vi "Transform_Calc_b_vector.vi"(9 "C":T1, 10 "PairedFiducialCoordinates":T2[](array[typedef]), 11 "A":T1) -> (3 "b":T1)   [LabVIEW 2011]
doc: "Coordinate system shift to transform reference point to the current coordinate system:\n\nY = A(X-C) + B \n\nWhere X is a point in the refernce system, C is the center of rotation offset to but the first fiducial at the origin for rotation, and A is the rotation and scaling matrix for the tranformation. Y is the coordinate for the point in the current coordinate system and this varialble B is the translation vector.\n\nThis should be approximately the (-1)*Fid_Current_Session(1), ie, the oposite sign of the shift to align the common fiducials for the rotation. Remember C is the shift for the reference session to do the same for it."
uses:
  <vilib>/Analysis/Matrix/Datatypes/RealMatrix.ctl
  Fiducial_pair.ctl
  <vilib>/Analysis/Matrix/Numeric/Conversions/Array To Matrix - RA.vi
  <vilib>/Analysis/Matrix/Numeric/Subtract/Subtract - RM,RM.vi
  <vilib>/Analysis/Matrix/Numeric/Multiply/Multiply - RM,RM.vi
  <vilib>/Analysis/Matrix/Numeric/Add/Add - RM,RM.vi
  <vilib>/Analysis/Matrix/NI_Matrix.lvlib
panel:
  out "A - B":dbl[][][](array[numeric])
  # "Fiducial Location Pair"
  # "Current Instrument Fiducial Location"
  # "Reference Instrument Fiducial Location"
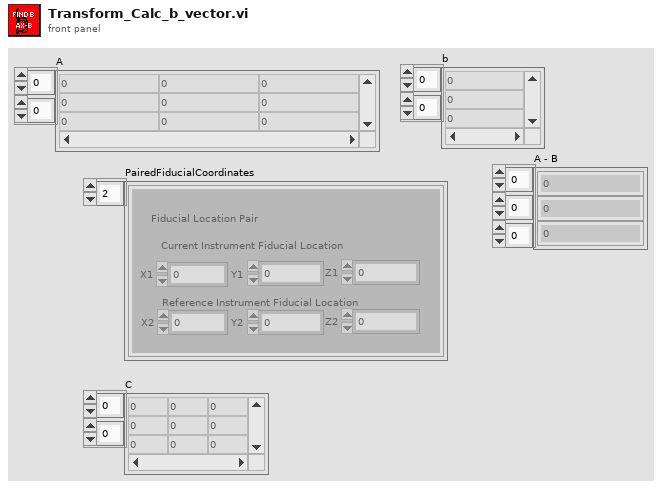
[diagram p1: front panel]
types:
  T1 = typedef "NI_Matrix.lvlib/RealMatrix.ctl" = dbl[][]
  T2 = typedef "Fiducial_pair.ctl" = cluster{"X1":dbl, "X2":dbl, "Y1":dbl, "Y2":dbl, "Z1":dbl, "Z2":dbl}
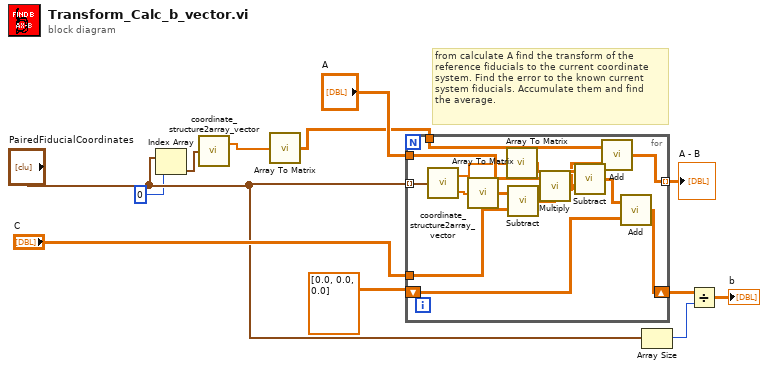
[diagram p0: block diagram]
diagram:
  # "from calculate A find the transform of the\nreference fiducials to the current coordinate\nsystem. Find the error to the known current \nsystem fiducials. Accumulate them and find\nthe average."
  n1 = Index Array(array="PairedFiducialCoordinates", index=0) -> (element=w3:T2)
  n2 = call "coordinate_structure2array_vector.vi"("Fiducial_Pos_structure"=w3) -> ("Current_Instrument_pos"=w2:dbl[])  [unwired: 1 out]
  n3 = call-poly <vilib>:"Array To Matrix.vi"("Real 1D Array"=w2) -> ("Real Matrix (Column Vector)"=w1:T1)
  n4 = for {
    tunnel: "A" -> [w26]
    shift-right: [w17] -> w8
    shift-left: T1 [[0.0], [0.0], [0.0]] ("A - B") -> [w24]
    tunnel: "PairedFiducialCoordinates" -> [w23] mode=indexing
    tunnel: "C" -> [w19]
    tunnel: [w13] -> w6 mode=indexing
    tunnel: w1 -> [w14]
    n5 = call "coordinate_structure2array_vector.vi"("Fiducial_Pos_structure"=w23) -> ("Current_Instrument_pos"=w22:dbl[], "Reference_Instrument_pos"=w21:dbl[])
    n6 = call-poly <vilib>:"Array To Matrix.vi"("Real 1D Array"=w21) -> ("Real Matrix (Column Vector)"=w20:T1)
    n7 = call-poly <vilib>:"Array To Matrix.vi"("Real 1D Array"=w22) -> ("Real Matrix (Column Vector)"=w25:T1)
    n8 = call-poly <vilib>:"Subtract.vi"("Real Matrix B"=w19, "Real Matrix A"=w20) -> ("A - B"=w18:T1)
    n9 = call-poly <vilib>:"Multiply.vi"("Real Matrix B"=w18, "Real Matrix A"=w26) -> ("A * B"=w15:T1)
    n10 = call-poly <vilib>:"Subtract.vi"("Real Matrix B"=w15, "Real Matrix A"=w25) -> ("A - B"=w16:T1)
    n11 = call-poly <vilib>:"Add.vi"("Real Matrix B"=w15, "Real Matrix A"=w14) -> ("A + B"=w13:T1)
    n12 = call-poly <vilib>:"Add.vi"("Real Matrix B"=w24, "Real Matrix A"=w16) -> ("A + B"=w17:T1)
  }
  "A - B" <- w6
  n13 = Array Size(array="PairedFiducialCoordinates") -> (size(s)=w9:i32)
  n14 = Divide(x=w8, y=w9) -> (x/y=→"b":T1)
